vi "Set Ref.vi"(4 "Name":string, 6 "Name Msg Strategy":string, 8 "error in":errorcluster, 9 "Name Library File Path":path, 10 "Project:Active Project":refnum<vi>) -> (0 "error out":errorcluster, 2 "Ref":T1)   [LabVIEW 2021, in "_Rescript Msg.lvlib" / "_Rescript Msg.lvclass"]
uses:
  _Rescript Msg.lvclass
  Ref.ctl
  <vilib>/Utility/traverseref.llb/TRef TravTarget.ctl
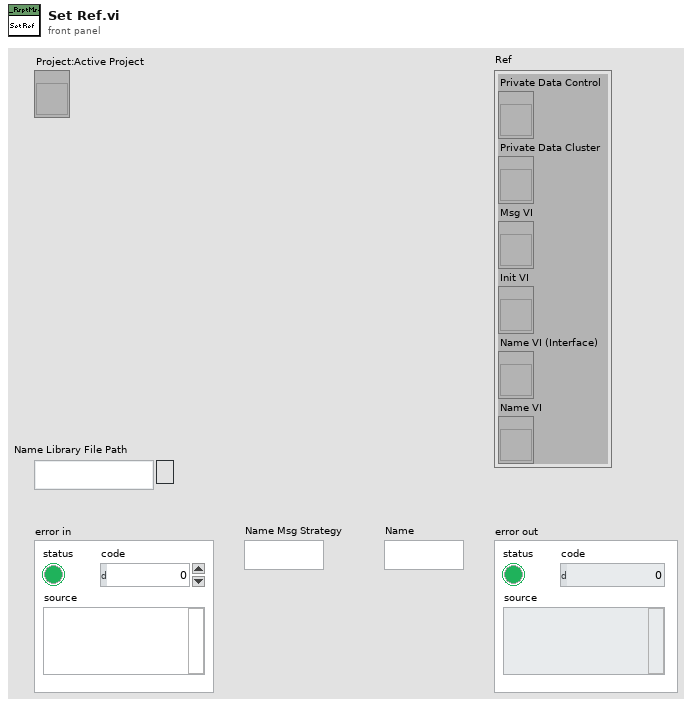
[diagram p1: front panel]
types:
  T1 = typedef "_Rescript Msg.lvlib/_Rescript Msg.lvclass/Ref.ctl" = cluster{"Private Data Control":refnum<vi>, "Private Data Cluster":refnum<vi>, "Msg VI":refnum<vi>, "Init VI":refnum<vi>, "Name VI (Interface)":refnum<vi>, "Name VI":refnum<vi>}
  T2 = typedef "TRef TravTarget.ctl" = enum16{"FP", "BD", "Other"}
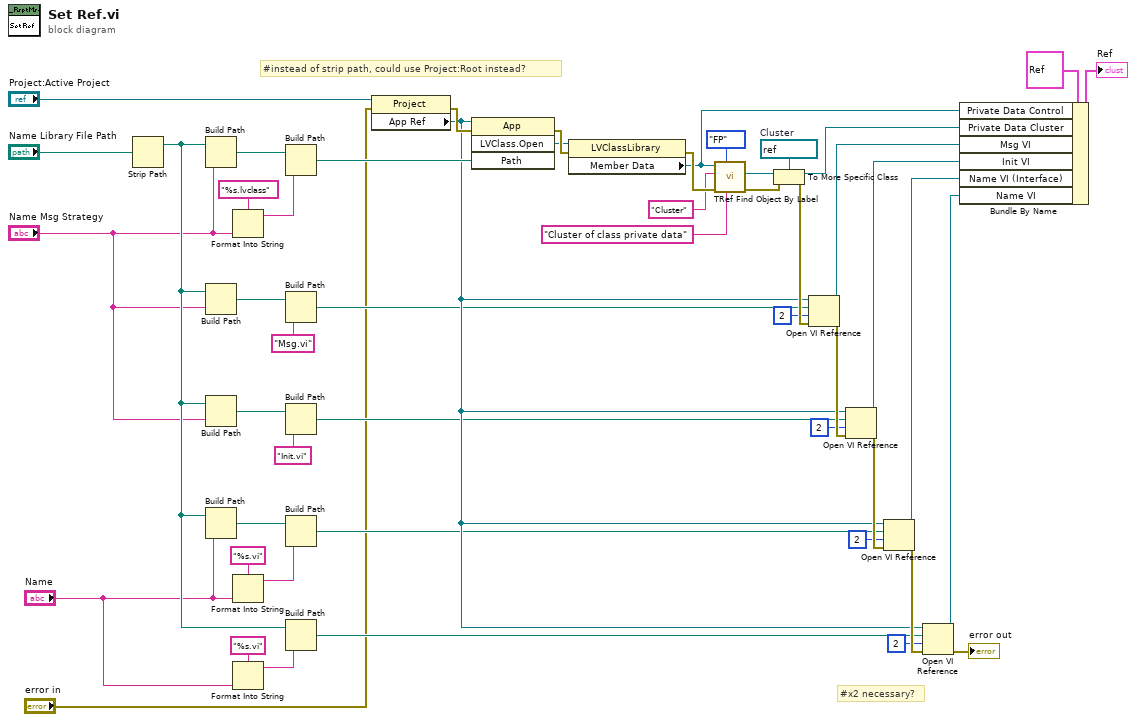
[diagram p0: block diagram]
diagram:
  w43 = refnum<vi> refnum  # Cluster
  # "#instead of strip path, could use Project:Root instead?"
  # "#x2 necessary?"
  n1 = Strip Path(path="Name Library File Path") -> (stripped path=w21:path)  [unwired: 1 out]
  n2 = Build Path(base path=w21, name or relative path="Name Msg Strategy") -> (appended path=w37:path)
  n3 = Build Path(base path=w21, name or relative path="Name Msg Strategy") -> (appended path=w29:path)
  n4 = Build Path(base path=w21, name or relative path="Name Msg Strategy") -> (appended path=w28:path)
  n5 = Build Path(base path=w21, name or relative path="Name") -> (appended path=w33:path)
  n6 = Format Into String(format string="%s.lvclass", "Name Msg Strategy") -> (resulting string=w35:string)  [unwired: 2 in, 1 out]
  n7 = Format Into String(format string="%s.vi", "Name") -> (resulting string=w32:string)  [unwired: 2 in, 1 out]
  n8 = Format Into String(format string="%s.vi", "Name") -> (resulting string=w22:string)  [unwired: 2 in, 1 out]
  n9 = Build Path(base path=w37, name or relative path=w35) -> (appended path=w36:path)
  n10 = Build Path(base path=w29, name or relative path="Msg.vi" ("format string")) -> (appended path=w25:path)
  n11 = Build Path(base path=w28, name or relative path="Init.vi" ("format string")) -> (appended path=w24:path)
  n12 = Build Path(base path=w33, name or relative path=w32) -> (appended path=w19:path)
  n13 = Build Path(base path=w21, name or relative path=w22) -> (appended path=w20:path)
  n14 = property class="Project"(reference="Project:Active Project", error in="error in") -> (error out=w47:errorcluster, "App Ref"=w30:refnum<vi>)  [unwired: 1 out]
  n15 = invoke class="App" method="LVClass.Open"(reference=w30, error in=w47, "Path"=w36) -> (error out=w45:errorcluster, "LVClass.Open"=w38:refnum<vi>)  [unwired: 1 in, 2 out]
  n16 = property class="LVClassLibrary"(reference=w38, error in=w45) -> (error out=w51:errorcluster, "Member Data"=w1:refnum<vi>)  [unwired: 1 out]
  n17 = call <vilib>:"TRef Find Object By Label.vi"("Label"="Cluster of class private data" ("Class Name"), "Traverse Target"=TRef_TravTarget."FP", "error in (no error)"=w51, "Class Name"="Cluster", "VI Ref"=w1) -> ("error out"=w44:errorcluster, "Found Obj Ref"=w42:refnum<vi>)  [unwired: 3 in, 2 out]
  n18 = To More Specific Class(target class=w43, reference=w42, error in=w44) -> (specific class reference=w6:refnum<vi>, error out=w46:errorcluster)
  n19 = Open VI Reference(application reference (local)=w30, vi path=w25, options=2, error in (no error)=w46) -> (vi reference=w7:refnum<vi>, error out=w50:errorcluster)  [unwired: 2 in]
  n20 = Open VI Reference(application reference (local)=w30, vi path=w24, options=2, error in (no error)=w50) -> (vi reference=w8:refnum<vi>, error out=w49:errorcluster)  [unwired: 2 in]
  n21 = Open VI Reference(application reference (local)=w30, vi path=w19, options=2, error in (no error)=w49) -> (vi reference=w9:refnum<vi>, error out=w48:errorcluster)  [unwired: 2 in]
  n22 = Open VI Reference(application reference (local)=w30, vi path=w20, options=2, error in (no error)=w48) -> (vi reference=w10:refnum<vi>, error out=→"error out":errorcluster)  [unwired: 2 in]
  n23 = Bundle By Name(cluster=T1 {"Private Data Control"=refnum, "Private Data Cluster"=refnum, "Msg VI"=refnum, "Init VI"=refnum, "Name VI (Interface)"=refnum, "Name VI"=refnum} ("Ref"), "Private Data Control"=w1, "Private Data Cluster"=w6, "Msg VI"=w7, "Init VI"=w8, "Name VI (Interface)"=w9, "Name VI"=w10) -> (→"Ref":T1)
